vi "Subpanel_Protected.vi"(7 "Autoshow? (T)":bool=TRUE, 8 "error in (no error)":errorcluster, 9 "Sub Panel":refnum<vi>, 11 "Subpanel in":refnum<class "Subpanel.lvclass">) -> (0 "error out":errorcluster, 3 "Subpanel out":refnum<class "Subpanel.lvclass">)   [LabVIEW 2023, in "Panel Actor.lvlib" / "Panel.lvlib" / "Subpanel.lvclass"]
doc: "A constructor that can be used by children of the subpanel class.\n\n----\nPlease see the following web address for additional documentation and tutorial information:\nhttp://www.mooregoodideas.com/mgi-panel-manager/\n\nAuthor: Derek Trepanier\n\nCopyright (c) 2018, Moore Good Ideas, Inc.\n\nAll rights reserved.\n\nRedistribution and use in source and binary forms, with or without modification, are permitted provided that the following conditions are met:\n\n * Redistributions of source code must retain the above copyright notice, this list of conditions and the following disclaimer.\n * Redistributions in binary form must reproduce the above copyright notice, this list of conditions and the following disclaimer in the documentation and/or other materials provided with the distribution.\n * Neither the name of Moore Good Ideas, Inc. nor the names of its contributors may be used to endorse or promote products derived from this software without specific prior written permission.\n\nTHIS SOFTWARE IS PROVIDED BY THE COPYRIGHT HOLDERS AND CONTRIBUTORS \"AS IS\" AND ANY EXPRESS OR IMPLIED WARRANTIES, INCLUDING, BUT NOT LIMITED TO, THE IMPLIED WARRANTIES OF MERCHANTABILITY AND FITNESS FOR A PARTICULAR PURPOSE ARE DISCLAIMED. IN NO EVENT SHALL THE COPYRIGHT OWNER OR CONTRIBUTORS BE LIABLE FOR ANY DIRECT, INDIRECT, INCIDENTAL, SPECIAL, EXEMPLARY, OR CONSEQUENTIAL DAMAGES (INCLUDING, BUT NOT LIMITED TO, PROCUREMENT OF SUBSTITUTE GOODS OR SERVICES; LOSS OF USE, DATA, OR PROFITS; OR BUSINESS INTERRUPTION) HOWEVER CAUSED AND ON ANY THEORY OF LIABILITY, WHETHER IN CONTRACT, STRICT LIABILITY, OR TORT (INCLUDING NEGLIGENCE OR OTHERWISE) ARISING IN ANY WAY OUT OF THE USE OF THIS SOFTWARE, EVEN IF ADVISED OF THE POSSIBILITY OF SUCH DAMAGE."
uses:
  Subpanel.lvclass
  Subpanel.lvclass/Subpanel.ctl
  Panel.lvclass
  Panel.lvlib
  C:/Users/Public/Documents/Development/Engine/Panel Manager/Panel/Panel/Panel.lvclass
  C:/Users/Public/Documents/Development/Engine/Panel Manager/Panel/Panel/Subpanel/Subpanel.lvclass
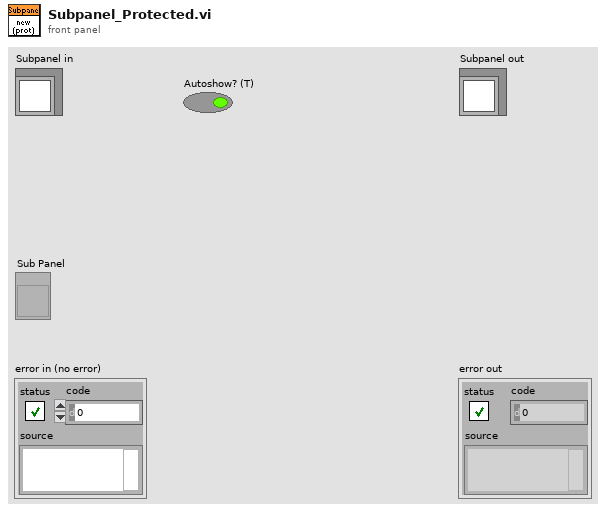
[diagram p1: front panel]
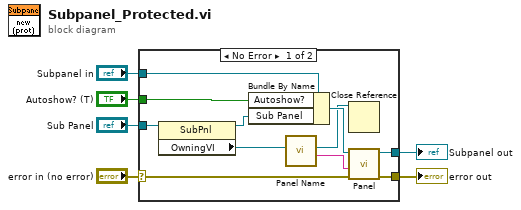
[diagram p0: block diagram]
diagram:
  n1 = case shown="No Error" "error in (no error)" {
    selector: "error in (no error)" -> [w13 w19]
    tunnel: [w14 w19] -> w2
    tunnel: [w15 w18] -> w3
    tunnel: "Subpanel in" -> [w17 w18]
    tunnel: "Sub Panel" -> [w12 _]
    tunnel: "Autoshow? (T)" -> [w10 _]
    frame No Error {
      n2 = property class="SubPnl"(reference=w12) -> (reference out=w11:refnum<vi>, "OwningVI"=w9:refnum<vi>)  [unwired: 1 in, 1 out]
      n3 = Bundle By Name(cluster=w17, "Autoshow?"=w10, "Sub Panel"=w11) -> (w16:refnum<class "Subpanel.lvclass">)
      n4 = call "Panel Name.vi"("VI in"=w9) -> ("Name"=w8:string, "VI out"=w7:refnum<vi>)  [unwired: 9 in]
      n5 = Close Reference(reference=w7) -> ()  [unwired: 1 in, 1 out]
      n6 = call "Panel.vi"("error in (no error)"=w13, "Parent Panel Name"=w8, "Panel in"=w16) -> ("error out"=w14:errorcluster, "Panel in"=w15:refnum<class "Subpanel.lvclass">)  [unwired: 7 in]
    }
    frame Error {
    }
  }
  "error out" <- w2
  "Subpanel out" <- w3
